vi "Plot Sine Graph with date & time.vi"() -> ()   [LabVIEW 2020]
uses:
  <vilib>/measure/NI_MABase.lvlib
panel:
  in  "stop":bool
  out "Waveform Chart":waveform(dbl)(graph)
  in  "Phase":dbl(knob) scale=0.0..180.0
  in  "Amplitude":dbl(knob) scale=0.0..10.0
  in  "Frequency":dbl(knob) scale=0.0..200.0
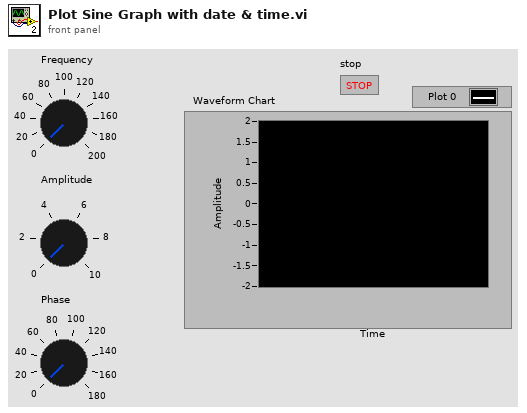
[diagram p1: front panel]
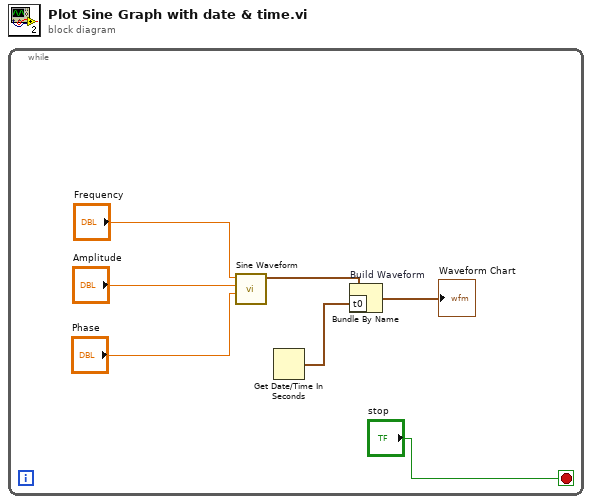
[diagram p0: block diagram]
diagram:
  n1 = while {
    stop <- "stop" stop-if-true
    n2 = call <vilib>:"Sine Waveform.vi"("phase"="Phase", "amplitude"="Amplitude", "frequency"="Frequency") -> ("signal out"=w4:waveform(dbl))  [unwired: 7 in, 1 out]
    n3 = Get Date/Time In Seconds() -> (seconds since 1Jan1904=w3:timestamp)
    n4 = Bundle By Name "Build Waveform"(cluster=w4, "t0"=w3) -> (→"Waveform Chart":waveform(dbl))
  }
